vi "Autonomous Independent.vi"   [LabVIEW 2015]
doc: "This VI is called when autonomous begins, and will automatically be terminated when autonomous ends. You can carry out timed or sensor driven robot movement independently without needing to return to the caller."
uses:
  Arm Mode TypeDef.ctl
  Global Variables.vi
panel:
  # "Be sure to right-click and choose Data Operations>>Make Current Value default if you want to save the array values with the VI"
types:
  T1 = typedef "IMU AHRS TypeDef.ctl" = cluster{"Pitch":dbl, "Roll":dbl, "Yaw":dbl}
  T2 = typedef "Autonomous Mode.ctl" = enum16{"Off", "Cross Defense", "Shoot A/B", "Shoot C/D", "Shoot E"}
  T3 = typedef "Arm Mode TypeDef.ctl" = enum16{"Unknown", "Disabled", "Locked", "Shoot Batter", "Shoot Close", "Cross Defense", "Human Player Load", "Low Bar / Goal", "Manual"}
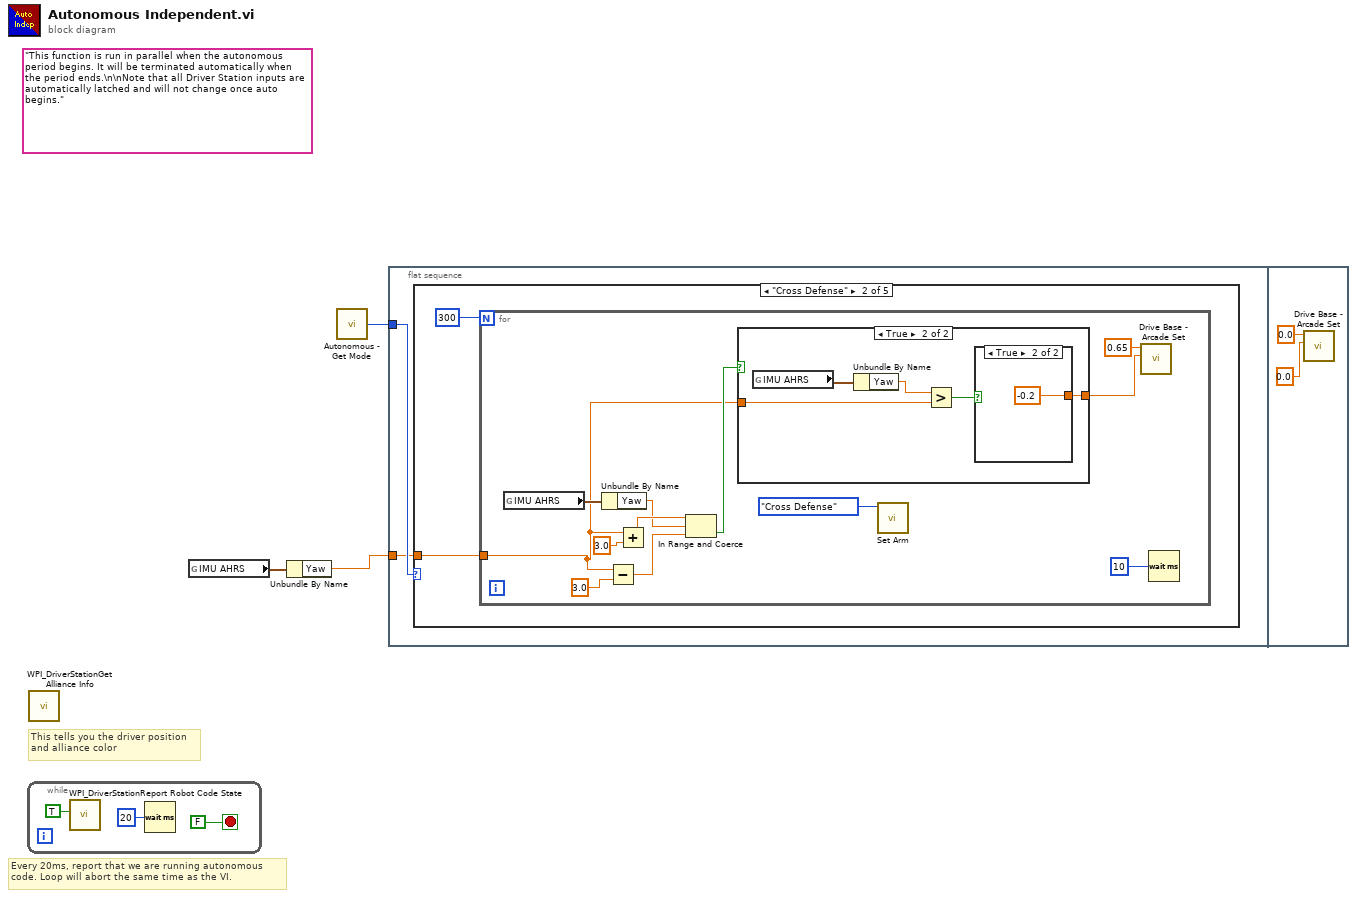
[diagram p0: block diagram]
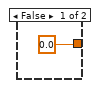
[diagram p3: hidden frame]
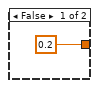
[diagram p4: hidden frame]
diagram:
  (unwired) "This function is run in parallel when the autonomous period begins. It will be terminated automatically when the period ends.\n\nNote that all Driver Station inputs are automatically latched and will not change once auto begins."
  # "Every 20ms, report that we are running autonomous\ncode. Loop will abort the same time as the VI."
  # "This tells you the driver position\nand alliance color"
  n1 = while {
    stop <- FALSE stop-if-true
    n2 = call <vilib>:"WPI_DriverStationReport Robot Code State.vi"("Autonomous"=TRUE) -> ()  [unwired: 10 in, 1 out]
    n3 = Wait (ms)(milliseconds to wait=u32 20) -> ()  [unwired: 1 out]
  }
  n4 = call <vilib>:"WPI_DriverStationGet Alliance Info.vi"() -> ()  [unwired: 12 out]
  n5 = global read "Global Variables.vi" "IMU AHRS"() -> (w2:T1)
  n6 = Unbundle By Name(w2) -> ("Yaw"=w1:dbl)
  n7 = call "Autonomous - Get Mode.vi"() -> ("Autonomous Mode"=w3:T2)  [unwired: 1 in]
  n8 = flat-sequence {
    tunnel: w3 -> [w8]
    tunnel: w1 -> [w7]
    frame #0 {
      n9 = case shown="\"Cross Defense\"" w8 {
        tunnel: w7 -> [_ w9 _ _ _]
        frame "Off", Default {
        }
        frame "Cross Defense" {
          n10 = for {
            N: 300 ("Numeric") -> [_]
            tunnel: w9 -> [w12]
            n11 = global read "Global Variables.vi" "IMU AHRS"() -> (w19:T1)
            n12 = Unbundle By Name(w19) -> ("Yaw"=w14:dbl)
            n13 = Subtract(x=w12, y=3.0) -> (x-y=w15:dbl)
            n14 = Add(x=w12, y=3.0) -> (x+y=w16:dbl)
            n15 = In Range and Coerce(upper limit=w16, x=w14, lower limit=w15) -> (In Range?=w13:bool)  [unwired: 1 out]
            n16 = case shown="True" w13 {
              tunnel: w12 -> [_ w25]
              tunnel: [0.0 w24] -> w11
              frame False {
              }
              frame True {
                n17 = global read "Global Variables.vi" "IMU AHRS"() -> (w26:T1)
                n18 = Unbundle By Name(w26) -> ("Yaw"=w27:dbl)
                n19 = Greater?(x=w27, y=w25) -> (0:w28:bool)
                n20 = case shown="True" w28 {
                  tunnel: [0.2 -0.2] -> w24
                  frame False {
                  }
                  frame True {
                  }
                }
              }
            }
            n21 = call "Set Arm.vi"("Arm Mode"=Arm_Mode_TypeDef."Cross Defense" ("Switch 3 Select")) -> ()  [unwired: 11 in]
            n22 = call "Drive Base - Arcade Set.vi"("X"=w11, "Y"=0.65) -> ()  [unwired: 9 in, 1 out]
            n23 = Wait (ms)(milliseconds to wait=u32 10) -> ()  [unwired: 1 out]
          }
        }
        frame "Shoot A/B" {
        }
        frame "Shoot C/D" {
        }
        frame "Shoot E" {
        }
      }
    }
    frame #1 {
      n24 = call "Drive Base - Arcade Set.vi"("X"=0.0, "Y"=0.0) -> ()  [unwired: 9 in, 1 out]
    }
  }
